vi "PH_Interaction.Open or Create PCS Instances.vi"(1 "System ID (N/A)":string="N/A", 2 "Instance to create or open":T1(ring), 5 "error IO":errorcluster) -> (19 "error out":errorcluster)   [LabVIEW 2014, in "PH_Common.lvlib"]
doc: "This VI reates or opens certain PCS Instances."
uses:
  PH_Common.lvlib
  CSCore/CSSystem/CSSystemLib/CSSystemLib.lvlib
  CSCore/CSObj/CSObj.lvlib
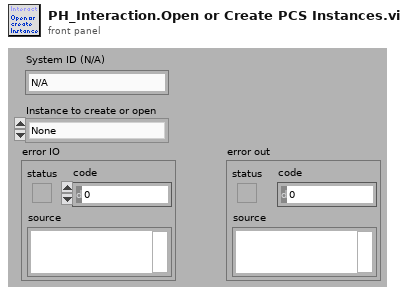
[diagram p1: front panel]
types:
  T1 = enum16{"None", "PCS Main", "Z6 Main", "PCS Beamline", "Z6 Beamline", "Image Statistician", "Powermeter Statistician", "SHS Anal Statistician", "Image Center of Gravity", "Image Calibrator", "SHS Analysis Calibrator", "Cam List", "Powermeterlist", "6P List", "BB List", "Switch List", "Sequence Watch"}
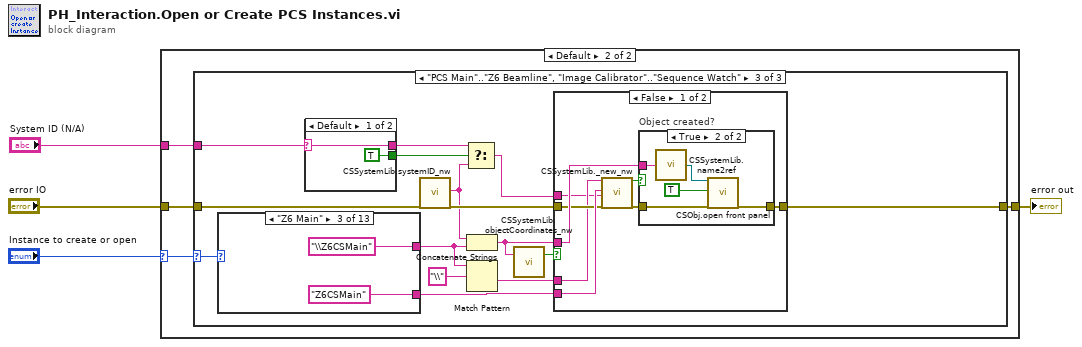
[diagram p0: block diagram]
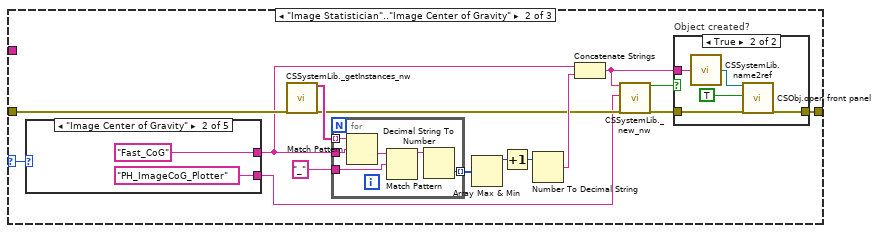
[diagram p4: hidden frame]
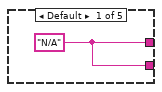
[diagram p6: hidden frame]
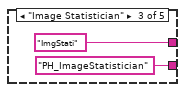
[diagram p7: hidden frame]
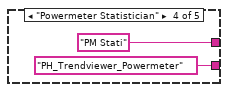
[diagram p8: hidden frame]
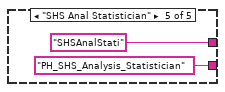
[diagram p9: hidden frame]
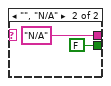
[diagram p10: hidden frame]
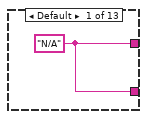
[diagram p11: hidden frame]
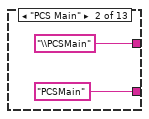
[diagram p12: hidden frame]
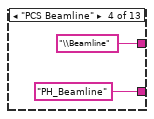
[diagram p13: hidden frame]
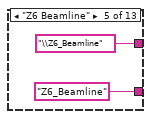
[diagram p14: hidden frame]
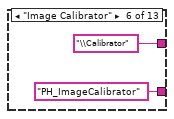
[diagram p15: hidden frame]
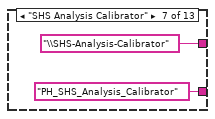
[diagram p16: hidden frame]
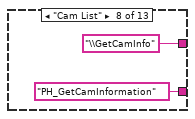
[diagram p17: hidden frame]
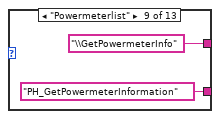
[diagram p18: hidden frame]
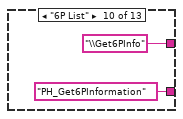
[diagram p19: hidden frame]
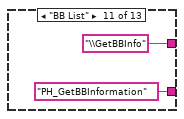
[diagram p20: hidden frame]
diagram:
  n1 = case shown="Default" "Instance to create or open" {
    selector: "Instance to create or open" -> [_ w8]
    tunnel: [w5 w7] -> w4
    tunnel: "error IO" -> [w5 w9]
    tunnel: "System ID (N/A)" -> [_ w6]
    frame "None" {
    }
    frame Default {
      n2 = case shown="\"PCS Main\"..\"Z6 Beamline\", \"Image Calibrator\"..\"Sequence Watch\"" w8 {
        selector: w8 -> [_ w17 w55]
        tunnel: [w10 w12 w57] -> w7
        tunnel: w9 -> [w10 w25 w56]
        tunnel: w6 -> [_ _ w49]
        frame Default {
        }
        frame "Image Statistician".."Image Center of Gravity" {
          n3 = case shown="\"Image Center of Gravity\"" w17 {
            tunnel: [w32 "PH_ImageCoG_Plotter" ("class name") "PH_ImageStatistician" ("class name") "PH_Trendviewer_Powermeter" ("class name") "PH_SHS_Analysis_Statistician" ("class name")] -> w11
            tunnel: [w32 "Fast_CoG" ("class name") "ImgStati" ("class name") "PM Stati" ("class name") "SHSAnalStati" ("class name")] -> w22
            frame Default {
              w32 = "N/A" ("class name")
            }
            frame "Image Center of Gravity" {
            }
            frame "Image Statistician" {
            }
            frame "Powermeter Statistician" {
            }
            frame "SHS Anal Statistician" {
            }
          }
          n4 = call "CSSystemLib._getInstances_nw.vi"("error in (no error)"=w25) -> ("i list"=w24:string[], "error out"=w13:errorcluster)  [unwired: 17 in]
          n5 = for {
            tunnel: w24 -> [w46] mode=indexing
            tunnel: w22 -> [w45]
            tunnel: "_" ("class name") -> [w44]
            tunnel: [w43] -> w19 mode=indexing
            n6 = Match Pattern(string=w46, regular expression=w45) -> (after substring=w42:string)  [unwired: 1 in, 3 out]
            n7 = Match Pattern(string=w42, regular expression=w44) -> (before substring=w41:string)  [unwired: 1 in, 3 out]
            n8 = Decimal String To Number(string=w41) -> (number=w43:i32)  [unwired: 2 in, 1 out]
          }
          n9 = Array Max & Min(array=w19) -> (max value=w20:i32)  [unwired: 3 out]
          n10 = Increment(x=w20) -> (x+1=w21:i32)
          n11 = Number To Decimal String(number=w21) -> (decimal integer string=w23:string)  [unwired: 1 in]
          n12 = Concatenate Strings(w22, w23) -> (w14:string)
          n13 = call "CSSystemLib._new_nw.vi"("objectName"=w14, "className"=w11, "error in (no error)"=w13) -> ("created new"=w15:bool, "error out"=w16:errorcluster)  [unwired: 14 in, 1 out]
          n14 = case "Object created?" shown="True" w15 {
            tunnel: [w26 w29] -> w12
            tunnel: w16 -> [w26 w31]
            tunnel: w14 -> [_ w28]
            frame False {
            }
            frame True {
              n15 = call "CSSystemLib.name2ref.vi"("name"=w28) -> ("obj refnum"=w27:refnum<vi>)
              n16 = call "CSObj.open front panel.vi"("i ref in"=w27, "frontPanelOpen"=TRUE ("front panel open"), "error in (no error)"=w31) -> ("error out"=w29:errorcluster)  [unwired: 15 in, 1 out]
            }
          }
        }
        frame "PCS Main".."Z6 Beamline", "Image Calibrator".."Sequence Watch" {
          n17 = case shown="\"Z6 Main\"" w55 {
            tunnel: [w66 "\\PCSMain" ("object name") "\\Z6CSMain" ("object name") "\\Beamline" ("object name") "\\Z6_Beamline" ("object name") "\\Calibrator" ("object name") "\\SHS-Analysis-Calibrator" ("object name") "\\GetCamInfo" ("object name") "\\GetPowermeterInfo" ("object name") "\\Get6PInfo" ("object name") "\\GetBBInfo" ("object name") "\\GetSwitchInfo" ("object name") "\\Sequencer-Info" ("object name")] -> w53
            tunnel: [w66 "PCSMain" ("class name") "Z6CSMain" ("class name") "PH_Beamline" ("class name") "Z6_Beamline" ("class name") "PH_ImageCalibrator" ("class name") "PH_SHS_Analysis_Calibrator" ("class name") "PH_GetCamInformation" ("class name") "PH_GetPowermeterInformation" ("class name") "PH_Get6PInformation" ("class name") "PH_GetBBInformation" ("class name") "PH_GetSwitchInformation" ("class name") "PH_Sequencer_Watch" ("class name")] -> w60
            frame Default {
              w66 = "N/A" ("object name")
            }
            frame "PCS Main" {
            }
            frame "Z6 Main" {
            }
            frame "PCS Beamline" {
            }
            frame "Z6 Beamline" {
            }
            frame "Image Calibrator" {
            }
            frame "SHS Analysis Calibrator" {
            }
            frame "Cam List" {
            }
            frame "Powermeterlist" {
            }
            frame "6P List" {
            }
            frame "BB List" {
            }
            frame "Switch List" {
            }
            frame "Sequence Watch" {
            }
          }
          n18 = case shown="Default" w49 {
            selector: w49 -> [w63 _]
            tunnel: [w63 "N/A"] -> w48
            tunnel: [TRUE FALSE] -> w47
            frame Default {
            }
            frame "", "N/A" {
            }
          }
          n19 = call "CSSystemLib.systemID_nw.vi"("error in (no error)"=w56) -> ("systemID out"=w51:string, "error out"=w61:errorcluster)  [unwired: 17 in]
          n20 = Select(t=w48, s=w47, f=w51) -> (s? t:f=w50:string)
          n21 = Concatenate Strings(w51, w53) -> (w59:string)
          n22 = Match Pattern(string=w53, regular expression="\\") -> (after substring=w52:string)  [unwired: 1 in, 3 out]
          n23 = call "CSSystemLib.objectCoordinates_nw.vi"("name"=w59) -> ("obj exists"=w58:bool)  [unwired: 15 in, 3 out]
          n24 = case shown="False" w58 {
            tunnel: [w93 w107] -> w57
            tunnel: w61 -> [w94 w108]
            tunnel: w60 -> [w96 _]
            tunnel: w59 -> [w95 w109]
            tunnel: w52 -> [w92 _]
            tunnel: w50 -> [w91 _]
            frame False {
              n25 = call "CSSystemLib._new_nw.vi"("objectName"=w92, "className"=w96, "systemName"=w91, "error in (no error)"=w94) -> ("created new"=w97:bool, "error out"=w98:errorcluster)  [unwired: 13 in, 1 out]
              n26 = case "Object created?" shown="True" w97 {
                tunnel: [w99 w102] -> w93
                tunnel: w98 -> [w99 w104]
                tunnel: w95 -> [_ w101]
                frame False {
                }
                frame True {
                  n27 = call "CSSystemLib.name2ref.vi"("name"=w101) -> ("obj refnum"=w100:refnum<vi>)
                  n28 = call "CSObj.open front panel.vi"("i ref in"=w100, "frontPanelOpen"=TRUE ("front panel open"), "error in (no error)"=w104) -> ("error out"=w102:errorcluster)  [unwired: 15 in, 1 out]
                }
              }
            }
            frame True {
              n29 = call "CSSystemLib.name2ref.vi"("name"=w109) -> ("obj refnum"=w106:refnum<vi>)
              n30 = call "CSObj.open front panel.vi"("i ref in"=w106, "frontPanelOpen"=TRUE ("front panel open"), "error in (no error)"=w108) -> ("error out"=w107:errorcluster)  [unwired: 15 in, 1 out]
            }
          }
        }
      }
    }
  }
  "error out" <- w4
